vi "nanocal -- nuclear schottky fit V7.vi"() -> ()   [LabVIEW 2021] (continued)
0.000047379208   ,  \"τC\" -> 0.003106112976   ,  \"κ0\" -> 0.000000012600   ,  \"mm1\" -> 0.000044370583   ,  \"mm2\" -> 0.017847763479   ,  \"mm3\" -> 0.023626714407   ,  \"T\" -> 1.900000000000   ,  \"B\" -> 6.000000000000   ,  \"θ\" -> 0.000000000000   ,  \"Reoff\" -> -371428.571428571827   ,  \"Imoff\" -> 0.000000000000   ,  \"στ1\" -> 0.007486573720   ,  \"στS\" -> 0.000328189496   ,  \"στN\" -> 0.000005492338    |>   , \n\"IDS0454_220529_RAW_cal__sam_\" ->   <|    \"ζ\" -> 0.000000000000   ,  \"τ1\" -> 0.000000000000   ,  \"τS\" -> 0.000000000000   ,  \"τN\" -> 0.000000000000   ,  \"τC\" -> 0.000000000000   ,  \"κ0\" -> 0.000000000000   ,  \"mm1\" -> 0.000000000000   ,  \"mm2\" -> 0.000000000000   ,  \"mm3\" -> 0.000000000000   ,  \"T\" -> 1.900000000000   ,  \"B\" -> 6.000000000000   ,  \"θ\" -> 0.000000000000   ,  \"Reoff\" -> 0.000000000000   ,  \"Imoff\" -> 0.000000000000   ,  \"στ1\" -> 0.000000000000   ,  \"στS\" -> 0.000000000000   ,  \"στN\" -> 0.000000000000    |>   , \n\"IDS0455_220529_RAW_cal__ref_\" ->   <|    \"ζ\" -> 0.017684542475   ,  \"τ1\" -> 0.025415252258   ,  \"τS\" -> 0.009236528363   ,  \"τN\" -> 0.000017905293   ,  \"τC\" -> 0.002401600721   ,  \"κ0\" -> 0.000000022300   ,  \"mm1\" -> 0.000033334613   ,  \"mm2\" -> 0.011752475280   ,  \"mm3\" -> 0.025449137167   ,  \"T\" -> 3.100000000000   ,  \"B\" -> 6.000000000000   ,  \"θ\" -> 0.000000000000   ,  \"Reoff\" -> -224489.795918366871   ,  \"Imoff\" -> 0.000000000000   ,  \"στ1\" -> 0.002319336344   ,  \"στS\" -> 0.000088789026   ,  \"στN\" -> 0.000000711840    |>   , \n\"IDS0455_220529_RAW_cal__sam_\" ->   <|    \"ζ\" -> 0.000000000000   ,  \"τ1\" -> 0.000000000000   ,  \"τS\" -> 0.000000000000   ,  \"τN\" -> 0.000000000000   ,  \"τC\" -> 0.000000000000   ,  \"κ0\" -> 0.000000000000   ,  \"mm1\" -> 0.000000000000   ,  \"mm2\" -> 0.000000000000   ,  \"mm3\" -> 0.000000000000   ,  \"T\" -> 3.100000000000   ,  \"B\" -> 6.000000000000   ,  \"θ\" -> 0.000000000000   ,  \"Reoff\" -> 0.000000000000   ,  \"Imoff\" -> 0.000000000000   ,  \"στ1\" -> 0.000000000000   ,  \"στS\" -> 0.000000000000   ,  \"στN\" -> 0.000000000000    |>   , \n\"IDS0456_220529_RAW_cal__ref_\" ->   <|    \"ζ\" -> 0.018735255997   ,  \"τ1\" -> 0.025807065758   ,  \"τS\" -> 0.005944253757   ,  \"τN\" -> 0.000004775198   ,  \"τC\" -> 0.001961268842   ,  \"κ0\" -> 0.000000054800   ,  \"mm1\" -> 0.000027338307   ,  \"mm2\" -> 0.007987373292   ,  \"mm3\" -> 0.025814108537   ,  \"T\" -> 5.700000000000   ,  \"B\" -> 6.000000000000   ,  \"θ\" -> 0.000000000000   ,  \"Reoff\" -> -77551.020408162847   ,  \"Imoff\" -> 0.000000000000   ,  \"στ1\" -> 0.003676288803   ,  \"στS\" -> 0.001284267534   ,  \"στN\" -> 0.000002465031    |>   , \n\"IDS0456_220529_RAW_cal__sam_\" ->   <|    \"ζ\" -> 0.000000000000   ,  \"τ1\" -> 0.000000000000   ,  \"τS\" -> 0.000000000000   ,  \"τN\" -> 0.000000000000   ,  \"τC\" -> 0.000000000000   ,  \"κ0\" -> 0.000000000000   ,  \"mm1\" -> 0.000000000000   ,  \"mm2\" -> 0.000000000000   ,  \"mm3\" -> 0.000000000000   ,  \"T\" -> 5.700000000000   ,  \"B\" -> 6.000000000000   ,  \"θ\" -> 0.000000000000   ,  \"Reoff\" -> 0.000000000000   ,  \"Imoff\" -> 0.000000000000   ,  \"στ1\" -> 0.000000000000   ,  \"στS\" -> 0.000000000000   ,  \"στN\" -> 0.000000000000    |>   , \n\"IDS0458_220529_RAW_cal__ref_\" ->   <|    \"ζ\" -> 0.271949590763   ,  \"τ1\" -> 0.082491161116   ,  \"τS\" -> 0.016634017124   ,  \"τN\" -> 0.004711774467   ,  \"τC\" -> 0.000759404494   ,  \"κ0\" -> 0.000000000880   ,  \"mm1\" -> 0.000157873787   ,  \"mm2\" -> 0.019859290085   ,  \"mm3\" -> 0.090384172617   ,  \"T\" -> 0.200000000000   ,  \"B\" -> 4.000000000000   ,  \"θ\" -> 0.000000000000   ,  \"Reoff\" -> -53755102.040816329400   ,  \"Imoff\" -> 0.000000000000   ,  \"στ1\" -> 0.009172162575   ,  \"στS\" -> 0.000087849728   ,  \"στN\" -> 0.000215184537    |>   , \n\"IDS0458_220529_RAW_cal__sam_\" ->   <|    \"ζ\" -> 0.000000000000   ,  \"τ1\" -> 0.000000000000   ,  \"τS\" -> 0.000000000000   ,  \"τN\" -> 0.000000000000   ,  \"τC\" -> 0.000000000000   ,  \"κ0\" -> 0.000000000000   ,  \"mm1\" -> 0.000000000000   ,  \"mm2\" -> 0.000000000000   ,  \"mm3\" -> 0.000000000000   ,  \"T\" -> 0.200000000000   ,  \"B\" -> 4.000000000000   ,  \"θ\" -> 0.000000000000   ,  \"Reoff\" -> 0.000000000000   ,  \"Imoff\" -> 0.000000000000   ,  \"στ1\" -> 0.000000000000   ,  \"στS\" -> 0.000000000000   ,  \"στN\" -> 0.000000000000    |>   , \n\"IDS0459_220529_RAW_cal__ref_\" ->   <|    \"ζ\" -> 0.169028221284   ,  \"τ1\" -> 0.092219125546   ,  \"τS\" -> 0.014617231308   ,  \"τN\" -> 0.003004665048   ,  \"τC\" -> 0.000894699791   ,  \"κ0\" -> 0.000000001215   ,  \"mm1\" -> 0.000123777676   ,  \"mm2\" -> 0.017061745572   ,  \"mm3\" -> 0.096528796242   ,  \"T\" -> 0.250000000000   ,  \"B\" -> 4.000000000000   ,  \"θ\" -> 0.000000000000   ,  \"Reoff\" -> -23428571.428571432800   ,  \"Imoff\" -> 0.000000000000   ,  \"στ1\" -> 0.009019898069   ,  \"στS\" -> 0.000072357815   ,  \"στN\" -> 0.000072194130    |>   , \n\"IDS0459_220529_RAW_cal__sam_\" ->   <|    \"ζ\" -> 0.000000000000   ,  \"τ1\" -> 0.000000000000   ,  \"τS\" -> 0.000000000000   ,  \"τN\" -> 0.000000000000   ,  \"τC\" -> 0.000000000000   ,  \"κ0\" -> 0.000000000000   ,  \"mm1\" -> 0.000000000000   ,  \"mm2\" -> 0.000000000000   ,  \"mm3\" -> 0.000000000000   ,  \"T\" -> 0.250000000000   ,  \"B\" -> 4.000000000000   ,  \"θ\" -> 0.000000000000   ,  \"Reoff\" -> 0.000000000000   ,  \"Imoff\" -> 0.000000000000   ,  \"στ1\" -> 0.000000000000   ,  \"στS\" -> 0.000000000000   ,  \"στN\" -> 0.000000000000    |>   , \n\"IDS0460_220529_RAW_cal__ref_\" ->   <|    \"ζ\" -> 0.121095025204   ,  \"τ1\" -> 0.101406294737   ,  \"τS\" -> 0.013797908139   ,  \"τN\" -> 0.002167085296   ,  \"τC\" -> 0.000940421698   ,  \"κ0\" -> 0.000000001550   ,  \"mm1\" -> 0.000096322687   ,  \"mm2\" -> 0.015862507367   ,  \"mm3\" -> 0.104286161098   ,  \"T\" -> 0.300000000000   ,  \"B\" -> 4.000000000000   ,  \"θ\" -> 0.000000000000   ,  \"Reoff\" -> -14857142.857142865700   ,  \"Imoff\" -> 0.000000000000   ,  \"στ1\" -> 0.003344660593   ,  \"στS\" -> 0.000083531617   ,  \"στN\" -> 0.000031930335    |>   , \n\"IDS0460_220529_RAW_cal__sam_\" ->   <|    \"ζ\" -> 0.000000000000   ,  \"τ1\" -> 0.000000000000   ,  \"τS\" -> 0.000000000000   ,  \"τN\" -> 0.000000000000   ,  \"τC\" -> 0.000000000000   ,  \"κ0\" -> 0.000000000000   ,  \"mm1\" -> 0.000000000000   ,  \"mm2\" -> 0.000000000000   ,  \"mm3\" -> 0.000000000000   ,  \"T\" -> 0.300000000000   ,  \"B\" -> 4.000000000000   ,  \"θ\" -> 0.000000000000   ,  \"Reoff\" -> 0.000000000000   ,  \"Imoff\" -> 0.000000000000   ,  \"στ1\" -> 0.000000000000   ,  \"στS\" -> 0.000000000000   ,  \"στN\" -> 0.000000000000    |>   , \n\"IDS0461_220529_RAW_cal__ref_\" ->   <|    \"ζ\" -> 0.088720032208   ,  \"τ1\" -> 0.108699367297   ,  \"τS\" -> 0.013278602208   ,  \"τN\" -> 0.001545664659   ,  \"τC\" -> 0.001067836739   ,  \"κ0\" -> 0.000000001950   ,  \"mm1\" -> 0.000081459775   ,  \"mm2\" -> 0.015170211659   ,  \"mm3\" -> 0.110655008903   ,  \"T\" -> 0.360000000000   ,  \"B\" -> 4.000000000000   ,  \"θ\" -> 0.000000000000   ,  \"Reoff\" -> -9714285.714285701520   ,  \"Imoff\" -> 0.000000000000   ,  \"στ1\" -> 0.011282789082   ,  \"στS\" -> 0.000097113540   ,  \"στN\" -> 0.000042096921    |>   , \n\"IDS0461_220529_RAW_cal__sam_\" ->   <|    \"ζ\" -> 0.000000000000   ,  \"τ1\" -> 0.000000000000   ,  \"τS\" -> 0.000000000000   ,  \"τN\" -> 0.000000000000   ,  \"τC\" -> 0.000000000000   ,  \"κ0\" -> 0.000000000000   ,  \"mm1\" -> 0.000000000000   ,  \"mm2\" -> 0.000000000000   ,  \"mm3\" -> 0.000000000000   ,  \"T\" -> 0.360000000000   ,  \"B\" -> 4.000000000000   ,  \"θ\" -> 0.000000000000   ,  \"Reoff\" -> 0.000000000000   ,  \"Imoff\" -> 0.000000000000   ,  \"στ1\" -> 0.000000000000   ,  \"στS\" -> 0.000000000000   ,  \"στN\" -> 0.000000000000    |>   , \n\"IDS0462_220530_RAW_cal__ref_\" ->   <|    \"ζ\" -> 0.343667501463   ,  \"τ1\" -> 0.112483041616   ,  \"τS\" -> 0.019628128809   ,  \"τN\" -> 0.010154591080   ,  \"τC\" -> 0.000829297605   ,  \"κ0\" -> 0.000000000715   ,  \"mm1\" -> 0.000207215692   ,  \"mm2\" -> 0.023410434838   ,  \"mm3\" -> 0.129712761510   ,  \"T\" -> 0.170000000000   ,  \"B\" -> 4.000000000000   ,  \"θ\" -> 0.000000000000   ,  \"Reoff\" -> -62857142.857142865700   ,  \"Imoff\" -> 0.000000000000   ,  \"στ1\" -> 0.089687632936   ,  \"στS\" -> 0.000139405002   ,  \"στN\" -> 0.005363489281    |>   , \n\"IDS0462_220530_RAW_cal__sam_\" ->   <|    \"ζ\" -> 0.000000000000   ,  \"τ1\" -> 0.000000000000   ,  \"τS\" -> 0.000000000000   ,  \"τN\" -> 0.000000000000   ,  \"τC\" -> 0.000000000000   ,  \"κ0\" -> 0.000000000000   ,  \"mm1\" -> 0.000000000000   ,  \"mm2\" -> 0.000000000000   ,  \"mm3\" -> 0.000000000000   ,  \"T\" -> 0.170000000000   ,  \"B\" -> 4.000000000000   ,  \"θ\" -> 0.000000000000   ,  \"Reoff\" -> 0.000000000000   ,  \"Imoff\" -> 0.000000000000   ,  \"στ1\" -> 0.000000000000   ,  \"στS\" -> 0.000000000000   ,  \"στN\" -> 0.000000000000    |>   , \n\"IDS0463_220530_RAW_cal__ref_\" ->   <|    \"ζ\" -> 0.430227807451   ,  \"τ1\" -> 0.103641258629   ,  \"τS\" -> 0.021841444015   ,  \"τN\" -> 0.013133276363   ,  \"τC\" -> 0.000817797243   ,  \"κ0\" -> 0.000000000620   ,  \"mm1\" -> 0.000241540150   ,  \"mm2\" -> 0.025640890482   ,  \"mm3\" -> 0.128598442882   ,  \"T\" -> 0.150000000000   ,  \"B\" -> 4.000000000000   ,  \"θ\" -> 0.000000000000   ,  \"Reoff\" -> -76204081.632653057600   ,  \"Imoff\" -> 0.000000000000   ,  \"στ1\" -> 0.056966109308   ,  \"στS\" -> 0.000433843322   ,  \"στN\" -> 0.005482906809    |>   , \n\"IDS0463_220530_RAW_cal__sam_\" ->   <|    \"ζ\" -> 0.000000000000   ,  \"τ1\" -> 0.000000000000   ,  \"τS\" -> 0.000000000000   ,  \"τN\" -> 0.000000000000   ,  \"τC\" -> 0.000000000000   ,  \"κ0\" -> 0.000000000000   ,  \"mm1\" -> 0.000000000000   ,  \"mm2\" -> 0.000000000000   ,  \"mm3\" -> 0.000000000000   ,  \"T\" -> 0.150000000000   ,  \"B\" -> 4.000000000000   ,  \"θ\" -> 0.000000000000   ,  \"Reoff\" -> 0.000000000000   ,  \"Imoff\" -> 0.000000000000   ,  \"στ1\" -> 0.000000000000   ,  \"στS\" -> 0.000000000000   ,  \"στN\" -> 0.000000000000    |>   , \n\"IDS0464_220530_RAW_cal__ref_\" ->   <|    \"ζ\" -> 0.675671528717   ,  \"τ1\" -> 0.134361338288   ,  \"τS\" -> 0.029407446025   ,  \"τN\" -> 0.029781674231   ,  \"τC\" -> 0.000802871531   ,  \"κ0\" -> 0.000000000450   ,  \"mm1\" -> 0.000320592060   ,  \"mm2\" -> 0.033310531198   ,  \"mm3\" -> 0.200714610183   ,  \"T\" -> 0.120000000000   ,  \"B\" -> 4.000000000000   ,  \"θ\" -> 0.000000000000   ,  \"Reoff\" -> -173428571.428571433000   ,  \"Imoff\" -> 0.000000000000   ,  \"στ1\" -> 0.117118369535   ,  \"στS\" -> 0.002310482505   ,  \"στN\" -> 0.019921704088    |>   , \n\"IDS0464_220530_RAW_cal__sam_\" ->   <|    \"ζ\" -> 0.000000000000   ,  \"τ1\" -> 0.000000000000   ,  \"τS\" -> 0.000000000000   ,  \"τN\" -> 0.000000000000   ,  \"τC\" -> 0.000000000000   ,  \"κ0\" -> 0.000000000000   ,  \"mm1\" -> 0.000000000000   ,  \"mm2\" -> 0.000000000000   ,  \"mm3\" -> 0.000000000000   ,  \"T\" -> 0.120000000000   ,  \"B\" -> 4.000000000000   ,  \"θ\" -> 0.000000000000   ,  \"Reoff\" -> 0.000000000000   ,  \"Imoff\" -> 0.000000000000   ,  \"στ1\" -> 0.000000000000   ,  \"στS\" -> 0.000000000000   ,  \"στN\" -> 0.000000000000    |>   , \n\"IDS0465_220530_RAW_cal__ref_\" ->   <|    \"ζ\" -> 0.065985765394   ,  \"τ1\" -> 0.113805435970   ,  \"τS\" -> 0.013450011184   ,  \"τN\" -> 0.001342731867   ,  \"τC\" -> 0.001243319385   ,  \"κ0\" -> 0.000000002410   ,  \"mm1\" -> 0.000071145975   ,  \"mm2\" -> 0.015287668803   ,  \"mm3\" -> 0.115458794101   ,  \"T\" -> 0.430000000000   ,  \"B\" -> 4.000000000000   ,  \"θ\" -> 0.000000000000   ,  \"Reoff\" -> -5918367.346938773990   ,  \"Imoff\" -> 0.000000000000   ,  \"στ1\" -> 0.012030942275   ,  \"στS\" -> 0.000092415308   ,  \"στN\" -> 0.000055296571    |>   , \n\"IDS0465_220530_RAW_cal__sam_\" ->   <|    \"ζ\" -> 0.000000000000   ,  \"τ1\" -> 0.000000000000   ,  \"τS\" -> 0.000000000000   ,  \"τN\" -> 0.000000000000   ,  \"τC\" -> 0.000000000000   ,  \"κ0\" -> 0.000000000000   ,  \"mm1\" -> 0.000000000000   ,  \"mm2\" -> 0.000000000000   ,  \"mm3\" -> 0.000000000000   ,  \"T\" -> 0.430000000000   ,  \"B\" -> 4.000000000000   ,  \"θ\" -> 0.000000000000   ,  \"Reoff\" -> 0.000000000000   ,  \"Imoff\" -> 0.000000000000   ,  \"στ1\" -> 0.000000000000   ,  \"στS\" -> 0.000000000000   ,  \"στN\" -> 0.000000000000    |>   , \n\"IDS0466_220530_RAW_cal__ref_\" ->   <|    \"ζ\" -> 0.050274873948   ,  \"τ1\" -> 0.117572813394   ,  \"τS\" -> 0.013965174353   ,  \"τN\" -> 0.000622498353   ,  \"τC\" -> 0.001752185729   ,  \"κ0\" -> 0.000000003045   ,  \"mm1\" -> 0.000075268427   ,  \"mm2\" -> 0.016239468880   ,  \"mm3\" -> 0.118331327928   ,  \"T\" -> 0.530000000000   ,  \"B\" -> 4.000000000000   ,  \"θ\" -> 0.000000000000   ,  \"Reoff\" -> -3204081.632653061300   ,  \"Imoff\" -> 0.000000000000   ,  \"στ1\" -> 0.009611649331   ,  \"στS\" -> 0.000172547734   ,  \"στN\" -> 0.000019241473    |>   , \n\"IDS0466_220530_RAW_cal__sam_\" ->   <|    \"ζ\" -> 0.000000000000   ,  \"τ1\" -> 0.000000000000   ,  \"τS\" -> 0.000000000000   ,  \"τN\" -> 0.000000000000   ,  \"τC\" -> 0.000000000000   ,  \"κ0\" -> 0.000000000000   ,  \"mm1\" -> 0.000000000000   ,  \"mm2\" -> 0.000000000000   ,  \"mm3\" -> 0.000000000000   ,  \"T\" -> 0.530000000000   ,  \"B\" -> 4.000000000000   ,  \"θ\" -> 0.000000000000   ,  \"Reoff\" -> 0.000000000000   ,  \"Imoff\" -> 0.000000000000   ,  \"στ1\" -> 0.000000000000   ,  \"στS\" -> 0.000000000000   ,  \"στN\" -> 0.000000000000    |>   , \n\"IDS0467_220530_RAW_cal__ref_\" ->   <|    \"ζ\" -> 0.041054990767   ,  \"τ1\" -> 0.119173098156   ,  \"τS\" -> 0.015405145420   ,  \"τN\" -> 0.000278319894   ,  \"τC\" -> 0.001789500233   ,  \"κ0\" -> 0.000000003708   ,  \"mm1\" -> 0.000063714353   ,  \"mm2\" -> 0.017712825393   ,  \"mm3\" -> 0.119513408481   ,  \"T\" -> 0.620000000000   ,  \"B\" -> 4.000000000000   ,  \"θ\" -> 0.000000000000   ,  \"Reoff\" -> -2755102.040816326160   ,  \"Imoff\" -> 0.000000000000   ,  \"στ1\" -> 0.018149556060   ,  \"στS\" -> 0.000211563346   ,  \"στN\" -> 0.000013374065    |>   , \n\"IDS0467_220530_RAW_cal__sam_\" ->   <|    \"ζ\" -> 0.000000000000   ,  \"τ1\" -> 0.000000000000   ,  \"τS\" -> 0.000000000000   ,  \"τN\" -> 0.000000000000   ,  \"τC\" -> 0.000000000000   ,  \"κ0\" -> 0.000000000000   ,  \"mm1\" -> 0.000000000000   ,  \"mm2\" -> 0.000000000000   ,  \"mm3\" -> 0.000000000000   ,  \"T\" -> 0.620000000000   ,  \"B\" -> 4.000000000000   ,  \"θ\" -> 0.000000000000   ,  \"Reoff\" -> 0.000000000000   ,  \"Imoff\" -> 0.000000000000   ,  \"στ1\" -> 0.000000000000   ,  \"στS\" -> 0.000000000000   ,  \"στN\" -> 0.000000000000    |>   , \n\"IDS0468_220530_RAW_cal__ref_\" ->   <|    \"ζ\" -> 0.028502781656   ,  \"τ1\" -> 0.123145264277   ,  \"τS\" -> 0.019280232525   ,  \"τN\" -> 0.000154237911   ,  \"τC\" -> 0.002123664207   ,  \"κ0\" -> 0.000000005085   ,  \"mm1\" -> 0.000053289074   ,  \"mm2\" -> 0.021865908006   ,  \"mm3\" -> 0.123338138308   ,  \"T\" -> 0.820000000000   ,  \"B\" -> 4.000000000000   ,  \"θ\" -> 0.000000000000   ,  \"Reoff\" -> -1265306.122448980810   ,  \"Imoff\" -> 0.000000000000   ,  \"στ1\" -> 0.018340702428   ,  \"στS\" -> 0.000185539060   ,  \"στN\" -> 0.000003670517    |>   , \n\"IDS0468_220530_RAW_cal__sam_\" ->   <|    \"ζ\" -> 0.000000000000   ,  \"τ1\" -> 0.000000000000   ,  \"τS\" -> 0.000000000000   ,  \"τN\" -> 0.000000000000   ,  \"τC\" -> 0.000000000000   ,  \"κ0\" -> 0.000000000000   ,  \"mm1\" -> 0.000000000000   ,  \"mm2\" -> 0.000000000000   ,  \"mm3\" -> 0.000000000000   ,  \"T\" -> 0.820000000000   ,  \"B\" -> 4.000000000000   ,  \"θ\" -> 0.000000000000   ,  \"Reoff\" -> 0.000000000000   ,  \"Imoff\" -> 0.000000000000   ,  \"στ1\" -> 0.000000000000   ,  \"στS\" -> 0.000000000000   ,  \"στN\" -> 0.000000000000    |>   , \n\"IDS0469_220530_RAW_cal__ref_\" ->   <|    \"ζ\" -> 0.021661724597   ,  \"τ1\" -> 0.135376034198   ,  \"τS\" -> 0.027370656195   ,  \"τN\" -> 0.000065416524   ,  \"τC\" -> 0.002262892828   ,  \"κ0\" -> 0.000000007163   ,  \"mm1\" -> 0.000044452306   ,  \"mm2\" -> 0.030162834530   ,  \"mm3\" -> 0.135462025560   ,  \"T\" -> 1.120000000000   ,  \"B\" -> 4.000000000000   ,  \"θ\" -> 0.000000000000   ,  \"Reoff\" -> -775510.204081632196   ,  \"Imoff\" -> 0.000000000000   ,  \"στ1\" -> 0.011862460543   ,  \"στS\" -> 0.000298822899   ,  \"στN\" -> 0.000002245413    |>   , \n\"IDS0469_220530_RAW_cal__sam_\" ->   <|    \"ζ\" -> 0.000000000000   ,  \"τ1\" -> 0.000000000000   ,  \"τS\" -> 0.000000000000   ,  \"τN\" -> 0.000000000000   ,  \"τC\" -> 0.000000000000   ,  \"κ0\" -> 0.000000000000   ,  \"mm1\" -> 0.000000000000   ,  \"mm2\" -> 0.000000000000   ,  \"mm3\" -> 0.000000000000   ,  \"T\" -> 1.120000000000   ,  \"B\" -> 4.000000000000   ,  \"θ\" -> 0.000000000000   ,  \"Reoff\" -> 0.000000000000   ,  \"Imoff\" -> 0.000000000000   ,  \"στ1\" -> 0.000000000000   ,  \"στS\" -> 0.000000000000   ,  \"στN\" -> 0.000000000000    |>   , \n\"IDS0470_220530_RAW_cal__ref_\" ->   <|    \"ζ\" -> 0.015441202200   ,  \"τ1\" -> 0.041977704334   ,  \"τS\" -> 0.036507196019   ,  \"τN\" -> 0.000016236903   ,  \"τC\" -> 0.002199544538   ,  \"κ0\" -> 0.000000012895   ,  \"mm1\" -> 0.000031599194   ,  \"mm2\" -> 0.039021251943   ,  \"mm3\" -> 0.042211796370   ,  \"T\" -> 1.900000000000   ,  \"B\" -> 4.000000000000   ,  \"θ\" -> 0.000000000000   ,  \"Reoff\" -> -265306.122448978945   ,  \"Imoff\" -> 0.000000000000   ,  \"στ1\" -> 0.036878491395   ,  \"στS\" -> 0.000608860312   ,  \"στN\" -> 0.000004645190    |>   , \n\"IDS0470_220530_RAW_cal__sam_\" ->   <|    \"ζ\" -> 0.000000000000   ,  \"τ1\" -> 0.000000000000   ,  \"τS\" -> 0.000000000000   ,  \"τN\" -> 0.000000000000   ,  \"τC\" -> 0.000000000000   ,  \"κ0\" -> 0.000000000000   ,  \"mm1\" -> 0.000000000000   ,  \"mm2\" -> 0.000000000000   ,  \"mm3\" -> 0.000000000000   ,  \"T\" -> 1.900000000000   ,  \"B\" -> 4.000000000000   ,  \"θ\" -> 0.000000000000   ,  \"Reoff\" -> 0.000000000000   ,  \"Imoff\" -> 0.000000000000   ,  \"στ1\" -> 0.000000000000   ,  \"στS\" -> 0.000000000000   ,  \"στN\" -> 0.000000000000    |>   , \n\"IDS0471_220530_RAW_cal__ref_\" ->   <|    \"ζ\" -> 0.014899977348   ,  \"τ1\" -> 0.039852327400   ,  \"τS\" -> 0.012042479771   ,  \"τN\" -> 0.000007668254   ,  \"τC\" -> 0.002248141599   ,  \"κ0\" -> 0.000000015723   ,  \"mm1\" -> 0.000027931492   ,  \"mm2\" -> 0.014437702970   ,  \"mm3\" -> 0.039864529495   ,  \"T\" -> 2.300000000000   ,  \"B\" -> 4.000000000000   ,  \"θ\" -> 0.000000000000   ,  \"Reoff\" -> -183673.469387754798   ,  \"Imoff\" -> 0.000000000000   ,  \"στ1\" -> 0.000774965788   ,  \"στS\" -> 0.000109876194   ,  \"στN\" -> 0.000000141932    |>   , \n\"IDS0471_220530_RAW_cal__sam_\" ->   <|    \"ζ\" -> 0.000000000000   ,  \"τ1\" -> 0.000000000000   ,  \"τS\" -> 0.000000000000   ,  \"τN\" -> 0.000000000000   ,  \"τC\" -> 0.000000000000   ,  \"κ0\" -> 0.000000000000   ,  \"mm1\" -> 0.000000000000   ,  \"mm2\" -> 0.000000000000   ,  \"mm3\" -> 0.000000000000   ,  \"T\" -> 2.300000000000   ,  \"B\" -> 4.000000000000   ,  \"θ\" -> 0.000000000000   ,  \"Reoff\" -> 0.000000000000   ,  \"Imoff\" -> 0.000000000000   ,  \"στ1\" -> 0.000000000000   ,  \"στS\" -> 0.000000000000   ,  \"στN\" -> 0.000000000000    |>   , \n\"IDS0472_220530_RAW_cal__ref_\" ->   <|    \"ζ\" -> 0.016604913016   ,  \"τ1\" -> 0.039295846672   ,  \"τS\" -> 0.009676137271   ,  \"τN\" -> 0.000004030512   ,  \"τC\" -> 0.002212920920   ,  \"κ0\" -> 0.000000022506   ,  \"mm1\" -> 0.000029579758   ,  \"mm2\" -> 0.012018345525   ,  \"mm3\" -> 0.039301748436   ,  \"T\" -> 3.070000000000   ,  \"B\" -> 4.000000000000   ,  \"θ\" -> 0.000000000000   ,  \"Reoff\" -> -183673.469387754798   ,  \"Imoff\" -> 0.000000000000   ,  \"στ1\" -> 0.024245559529   ,  \"στS\" -> 0.008314224018   ,  \"στN\" -> 0.000009266489    |>   , \n\"IDS0472_220530_RAW_cal__sam_\" ->   <|    \"ζ\" -> 0.000000000000   ,  \"τ1\" -> 0.000000000000   ,  \"τS\" -> 0.000000000000   ,  \"τN\" -> 0.000000000000   ,  \"τC\" -> 0.000000000000   ,  \"κ0\" -> 0.000000000000   ,  \"mm1\" -> 0.000000000000   ,  \"mm2\" -> 0.000000000000   ,  \"mm3\" -> 0.000000000000   ,  \"T\" -> 3.070000000000   ,  \"B\" -> 4.000000000000   ,  \"θ\" -> 0.000000000000   ,  \"Reoff\" -> 0.000000000000   ,  \"Imoff\" -> 0.000000000000   ,  \"στ1\" -> 0.000000000000   ,  \"στS\" -> 0.000000000000   ,  \"στN\" -> 0.000000000000    |>   , \n\"IDS0473_220531_RAW_cal__ref_\" ->   <|    \"ζ\" -> 0.018700689738   ,  \"τ1\" -> 0.039247142341   ,  \"τS\" -> 0.006094502124   ,  \"τN\" -> 0.000001379348   ,  \"τC\" -> 0.001765569741   ,  \"κ0\" -> 0.000000055137   ,  \"mm1\" -> 0.000025315301   ,  \"mm2\" -> 0.007948371438   ,  \"mm3\" -> 0.039248904003   ,  \"T\" -> 5.700000000000   ,  \"B\" -> 4.000000000000   ,  \"θ\" -> 0.000000000000   ,  \"Reoff\" -> -102040.816326530650   ,  \"Imoff\" -> 0.000000000000   ,  \"στ1\" -> 0.006123782667   ,  \"στS\" -> 0.001309533453   ,  \"στN\" -> 0.000000787923    |>   , \n\"IDS0473_220531_RAW_cal__sam_\" ->   <|    \"ζ\" -> 0.000000000000   ,  \"τ1\" -> 0.000000000000   ,  \"τS\" -> 0.000000000000   ,  \"τN\" -> 0.000000000000   ,  \"τC\" -> 0.000000000000   ,  \"κ0\" -> 0.000000000000   ,  \"mm1\" -> 0.000000000000   ,  \"mm2\" -> 0.000000000000   ,  \"mm3\" -> 0.000000000000   ,  \"T\" -> 5.700000000000   ,  \"B\" -> 4.000000000000   ,  \"θ\" -> 0.000000000000   ,  \"Reoff\" -> 0.000000000000   ,  \"Imoff\" -> 0.000000000000   ,  \"στ1\" -> 0.000000000000   ,  \"στS\" -> 0.000000000000   ,  \"στN\" -> 0.000000000000    |>   , \n\"IDS0477_220601_RAW_cal__ref_\" ->   <|    \"ζ\" -> 0.239805642697   ,  \"τ1\" -> 0.033790664831   ,  \"τS\" -> 0.059024379220   ,  \"τN\" -> 0.060427064379   ,  \"τC\" -> 0.000896937980   ,  \"κ0\" -> 0.000000000920   ,  \"mm1\" -> 0.000171776345   ,  \"mm2\" -> 0.014890032084   ,  \"mm3\" -> 0.167722368184   ,  \"T\" -> 0.200000000000   ,  \"B\" -> 10.000000000000   ,  \"θ\" -> 45.000000000000   ,  \"Reoff\" -> -36122448.979591839000   ,  \"Imoff\" -> 0.000000000000   ,  \"στ1\" -> 0.011907202865   ,  \"στS\" -> 0.006392080806   ,  \"στN\" -> 0.010956766376    |>   , \n\"IDS0477_220601_RAW_cal__sam_\" ->   <|    \"ζ\" -> 0.000000000000   ,  \"τ1\" -> 0.000000000000   ,  \"τS\" -> 0.000000000000   ,  \"τN\" -> 0.000000000000   ,  \"τC\" -> 0.000000000000   ,  \"κ0\" -> 0.000000000000   ,  \"mm1\" -> 0.000000000000   ,  \"mm2\" -> 0.000000000000   ,  \"mm3\" -> 0.000000000000   ,  \"T\" -> 0.200000000000   ,  \"B\" -> 10.000000000000   ,  \"θ\" -> 45.000000000000   ,  \"Reoff\" -> 0.000000000000   ,  \"Imoff\" -> 0.000000000000   ,  \"στ1\" -> 0.000000000000   ,  \"στS\" -> 0.000000000000   ,  \"στN\" -> 0.000000000000    |>   , \n\"IDS0478_220601_RAW_cal__ref_\" ->   <|    \"ζ\" -> 0.152803180528   ,  \"τ1\" -> 0.028187868792   ,  \"τS\" -> 0.047098340694   ,  \"τN\" -> 0.025207837056   ,  \"τC\" -> 0.000982024605   ,  \"κ0\" -> 0.000000001260   ,  \"mm1\" -> 0.000128146365   ,  \"mm2\" -> 0.016152622122   ,  \"mm3\" -> 0.096243916593   ,  \"T\" -> 0.250000000000   ,  \"B\" -> 10.000000000000   ,  \"θ\" -> 45.000000000000   ,  \"Reoff\" -> -18163265.306122452000   ,  \"Imoff\" -> 0.000000000000   ,  \"στ1\" -> 0.005041045857   ,  \"στS\" -> 0.001567344139   ,  \"στN\" -> 0.002277988599    |>   , \n\"IDS0478_220601_RAW_cal__sam_\" ->   <|    \"ζ\" -> 0.000000000000   ,  \"τ1\" -> 0.000000000000   ,  \"τS\" -> 0.000000000000   ,  \"τN\" -> 0.000000000000   ,  \"τC\" -> 0.000000000000   ,  \"κ0\" -> 0.000000000000   ,  \"mm1\" -> 0.000000000000   ,  \"mm2\" -> 0.000000000000   ,  \"mm3\" -> 0.000000000000   ,  \"T\" -> 0.250000000000   ,  \"B\" -> 10.000000000000   ,  \"θ\" -> 45.000000000000   ,  \"Reoff\" -> 0.000000000000   ,  \"Imoff\" -> 0.000000000000   ,  \"στ1\" -> 0.000000000000   ,  \"στS\" -> 0.000000000000   ,  \"στN\" -> 0.000000000000    |>   , \n\"IDS0479_220601_RAW_cal__ref_\" ->   <|    \"ζ\" -> 0.111193066205   ,  \"τ1\" -> 0.024122553376   ,  \"τS\" -> 0.042118651402   ,  \"τN\" -> 0.013651970206   ,  \"τC\" -> 0.001072327817   ,  \"κ0\" -> 0.000000001570   ,  \"mm1\" -> 0.000105128315   ,  \"mm2\" -> 0.016280391263   ,  \"mm3\" -> 0.070781289644   ,  \"T\" -> 0.300000000000   ,  \"B\" -> 10.000000000000   ,  \"θ\" -> 45.000000000000   ,  \"Reoff\" -> -10816326.530612245200   ,  \"Imoff\" -> 0.000000000000   ,  \"στ1\" -> 0.003531051170   ,  \"στS\" -> 0.000678989919   ,  \"στN\" -> 0.000877996668    |>   , \n\"IDS0479_220601_RAW_cal__sam_\" ->   <|    \"ζ\" -> 0.000000000000   ,  \"τ1\" -> 0.000000000000   ,  \"τS\" -> 0.000000000000   ,  \"τN\" -> 0.000000000000   ,  \"τC\" -> 0.000000000000   ,  \"κ0\" -> 0.000000000000   ,  \"mm1\" -> 0.000000000000   ,  \"mm2\" -> 0.000000000000   ,  \"mm3\" -> 0.000000000000   ,  \"T\" -> 0.300000000000   ,  \"B\" -> 10.000000000000   ,  \"θ\" -> 45.000000000000   ,  \"Reoff\" -> 0.000000000000   ,  \"Imoff\" -> 0.000000000000   ,  \"στ1\" -> 0.000000000000   ,  \"στS\" -> 0.000000000000   ,  \"στN\" -> 0.000000000000    |>   , \n\"IDS0480_220601_RAW_cal__ref_\" ->   <|    \"ζ\" -> 0.079231560459   ,  \"τ1\" -> 0.017107381840   ,  \"τS\" -> 0.036891145607   ,  \"τN\" -> 0.007202328301   ,  \"τC\" -> 0.001264563258   ,  \"κ0\" -> 0.000000002000   ,  \"mm1\" -> 0.000090175019   ,  \"mm2\" -> 0.013352548983   ,  \"mm3\" -> 0.052516289748   ,  \"T\" -> 0.360000000000   ,  \"B\" -> 10.000000000000   ,  \"θ\" -> 45.000000000000   ,  \"Reoff\" -> -6326530.612244904040   ,  \"Imoff\" -> 0.000000000000   ,  \"στ1\" -> 0.001933309697   ,  \"στS\" -> 0.000284795622   ,  \"στN\" -> 0.000344056722    |>   , \n\"IDS0480_220601_RAW_cal__sam_\" ->   <|    \"ζ\" -> 0.000000000000   ,  \"τ1\" -> 0.000000000000   ,  \"τS\" -> 0.000000000000   ,  \"τN\" -> 0.000000000000   ,  \"τC\" -> 0.000000000000   ,  \"κ0\" -> 0.000000000000   ,  \"mm1\" -> 0.000000000000   ,  \"mm2\" -> 0.000000000000   ,  \"mm3\" -> 0.000000000000   ,  \"T\" -> 0.360000000000   ,  \"B\" -> 10.000000000000   ,  \"θ\" -> 45.000000000000   ,  \"Reoff\" -> 0.000000000000   ,  \"Imoff\" -> 0.000000000000   ,  \"στ1\" -> 0.000000000000   ,  \"στS\" -> 0.000000000000   ,  \"στN\" -> 0.000000000000    |>   , \n\"IDS0481_220601_RAW_cal__ref_\" ->   <|    \"ζ\" -> 0.059346185114   ,  \"τ1\" -> 0.015969775027   ,  \"τS\" -> 0.034144098652   ,  \"τN\" -> 0.004294468384   ,  \"τC\" -> 0.001604549811   ,  \"κ0\" -> 0.000000002410   ,  \"mm1\" -> 0.000086265768   ,  \"mm2\" -> 0.013446939913   ,  \"mm3\" -> 0.044760868507   ,  \"T\" -> 0.420000000000   ,  \"B\" -> 10.000000000000   ,  \"θ\" -> 45.000000000000   ,  \"Reoff\" -> -3061224.489795923230   ,  \"Imoff\" -> 0.000000000000   ,  \"στ1\" -> 0.000907344416   ,  \"στS\" -> 0.000176030005   ,  \"στN\" -> 0.000148751487    |>   , \n\"IDS0481_220601_RAW_cal__sam_\" ->   <|    \"ζ\" -> 0.000000000000   ,  \"τ1\" -> 0.000000000000   ,  \"τS\" -> 0.000000000000   ,  \"τN\" -> 0.000000000000   ,  \"τC\" -> 0.000000000000   ,  \"κ0\" -> 0.000000000000   ,  \"mm1\" -> 0.000000000000   ,  \"mm2\" -> 0.000000000000   ,  \"mm3\" -> 0.000000000000   ,  \"T\" -> 0.420000000000   ,  \"B\" -> 10.000000000000   ,  \"θ\" -> 45.000000000000   ,  \"Reoff\" -> 0.000000000000   ,  \"Imoff\" -> 0.000000000000   ,  \"στ1\" -> 0.000000000000   ,  \"στS\" -> 0.000000000000   ,  \"στN\" -> 0.000000000000    |>   , \n\"IDS0482_220601_RAW_cal__ref_\" ->   <|    \"ζ\" -> 0.043142553496   ,  \"τ1\" -> 0.014499389185   ,  \"τS\" -> 0.030371945733   ,  \"τN\" -> 0.002402650316   ,  \"τC\" -> 0.001877907190   ,  \"κ0\" -> 0.000000003100   ,  \"mm1\" -> 0.000073480289   ,  \"mm2\" -> 0.012924539137   ,  \"mm3\" -> 0.037567852762   ,  \"T\" -> 0.520000000000   ,  \"B\" -> 10.000000000000   ,  \"θ\" -> 45.000000000000   ,  \"Reoff\" -> -1836734.693877555430   ,  \"Imoff\" -> 0.000000000000   ,  \"στ1\" -> 0.000488095502   ,  \"στS\" -> 0.000097405917   ,  \"στN\" -> 0.000051506778    |>   , \n\"IDS0482_220601_RAW_cal__sam_\" ->   <|    \"ζ\" -> 0.000000000000   ,  \"τ1\" -> 0.000000000000   ,  \"τS\" -> 0.000000000000   ,  \"τN\" -> 0.000000000000   ,  \"τC\" -> 0.000000000000   ,  \"κ0\" -> 0.000000000000   ,  \"mm1\" -> 0.000000000000   ,  \"mm2\" -> 0.000000000000   ,  \"mm3\" -> 0.000000000000   ,  \"T\" -> 0.520000000000   ,  \"B\" -> 10.000000000000   ,  \"θ\" -> 45.000000000000   ,  \"Reoff\" -> 0.000000000000   ,  \"Imoff\" -> 0.000000000000   ,  \"στ1\" -> 0.000000000000   ,  \"στS\" -> 0.000000000000   ,  \"στN\" -> 0.000000000000    |>   , \n\"IDS0483_220601_RAW_cal__ref_\" ->   <|    \"ζ\" -> 0.037957534412   ,  \"τ1\" -> 0.013025982486   ,  \"τS\" -> 0.027861955043   ,  \"τN\" -> 0.001482537125   ,  \"τC\" -> 0.001562153050   ,  \"κ0\" -> 0.000000003750   ,  \"mm1\" -> 0.000054295490   ,  \"mm2\" -> 0.012021211304   ,  \"mm3\" -> 0.032970965481   ,  \"T\" -> 0.620000000000   ,  \"B\" -> 10.000000000000   ,  \"θ\" -> 45.000000000000   ,  \"Reoff\" -> -2489795.918367348610   ,  \"Imoff\" -> 0.000000000000   ,  \"στ1\" -> 0.000872811735   ,  \"στS\" -> 0.000114206450   ,  \"στN\" -> 0.000055407234    |>   , \n\"IDS0483_220601_RAW_cal__sam_\" ->   <|    \"ζ\" -> 0.000000000000   ,  \"τ1\" -> 0.000000000000   ,  \"τS\" -> 0.000000000000   ,  \"τN\" -> 0.000000000000   ,  \"τC\" -> 0.000000000000   ,  \"κ0\" -> 0.000000000000   ,  \"mm1\" -> 0.000000000000   ,  \"mm2\" -> 0.000000000000   ,  \"mm3\" -> 0.000000000000   ,  \"T\" -> 0.620000000000   ,  \"B\" -> 10.000000000000   ,  \"θ\" -> 45.000000000000   ,  \"Reoff\" -> 0.000000000000   ,  \"Imoff\" -> 0.000000000000   ,  \"στ1\" -> 0.000000000000   ,  \"στS\" -> 0.000000000000   ,  \"στN\" -> 0.000000000000    |>   , \n\"IDS0484_220601_RAW_cal__ref_\" ->   <|    \"ζ\" -> 0.026779879048   ,  \"τ1\" -> 0.012724854717   ,  \"τS\" -> 0.023406495826   ,  \"τN\" -> 0.000845574693   ,  \"τC\" -> 0.002190018434   ,  \"κ0\" -> 0.000000005114   ,  \"mm1\" -> 0.000052452848   ,  \"mm2\" -> 0.011990951083   ,  \"mm3\" -> 0.027773007254   ,  \"T\" -> 0.820000000000   ,  \"B\" -> 10.000000000000   ,  \"θ\" -> 45.000000000000   ,  \"Reoff\" -> -1020408.163265310230   ,  \"Imoff\" -> 0.000000000000   ,  \"στ1\" -> 0.000585844678   ,  \"στS\" -> 0.000123901377   ,  \"στN\" -> 0.000022627070    |>   , \n\"IDS0484_220601_RAW_cal__sam_\" ->   <|    \"ζ\" -> 0.000000000000   ,  \"τ1\" -> 0.000000000000   ,  \"τS\" -> 0.000000000000   ,  \"τN\" -> 0.000000000000   ,  \"τC\" -> 0.000000000000   ,  \"κ0\" -> 0.000000000000   ,  \"mm1\" -> 0.000000000000   ,  \"mm2\" -> 0.000000000000   ,  \"mm3\" -> 0.000000000000   ,  \"T\" -> 0.820000000000   ,  \"B\" -> 10.000000000000   ,  \"θ\" -> 45.000000000000   ,  \"Reoff\" -> 0.000000000000   ,  \"Imoff\" -> 0.000000000000   ,  \"στ1\" -> 0.000000000000   ,  \"στS\" -> 0.000000000000   ,  \"στN\" -> 0.000000000000    |>   , \n\"IDS0485_220601_RAW_cal__ref_\" ->   <|    \"ζ\" -> 0.326622885443   ,  \"τ1\" -> 0.044212332753   ,  \"τS\" -> 0.078119393187   ,  \"τN\" -> 0.109436103453   ,  \"τC\" -> 0.000856629079   ,  \"κ0\" -> 0.000000000725   ,  \"mm1\" -> 0.000209590105   ,  \"mm2\" -> 0.016643396508   ,  \"mm3\" -> 0.277031389353   ,  \"T\" -> 0.170000000000   ,  \"B\" -> 10.000000000000   ,  \"θ\" -> 45.000000000000   ,  \"Reoff\" -> -62040816.326530613000   ,  \"Imoff\" -> 0.000000000000   ,  \"στ1\" -> 0.024054965225   ,  \"στS\" -> 0.017110063636   ,  \"στN\" -> 0.032486922745    |>   , \n\"IDS0485_220601_RAW_cal__sam_\" ->   <|    \"ζ\" -> 0.000000000000   ,  \"τ1\" -> 0.000000000000   ,  \"τS\" -> 0.000000000000   ,  \"τN\" -> 0.000000000000   ,  \"τC\" -> 0.000000000000   ,  \"κ0\" -> 0.000000000000   ,  \"mm1\" -> 0.000000000000   ,  \"mm2\" -> 0.000000000000   ,  \"mm3\" -> 0.000000000000   ,  \"T\" -> 0.170000000000   ,  \"B\" -> 10.000000000000   ,  \"θ\" -> 45.000000000000   ,  \"Reoff\" -> 0.000000000000   ,  \"Imoff\" -> 0.000000000000   ,  \"στ1\" -> 0.000000000000   ,  \"στS\" -> 0.000000000000   ,  \"στN\" -> 0.000000000000    |>   , \n\"IDS0486_220602_RAW_cal__ref_\" ->   <|    \"ζ\" -> 0.647357967210   ,  \"τ1\" -> 0.057848718155   ,  \"τS\" -> 0.135216834392   ,  \"τN\" -> 0.439833290844   ,  \"τC\" -> 0.000803496040   ,  \"κ0\" -> 0.000000000457   ,  \"mm1\" -> 0.000315044381   ,  \"mm2\" -> 0.013010354662   ,  \"mm3\" -> 0.992640220504   ,  \"T\" -> 0.120000000000   ,  \"B\" -> 10.000000000000   ,  \"θ\" -> 45.000000000000   ,  \"Reoff\" -> -171836734.693877578000   ,  \"Imoff\" -> 0.000000000000   ,  \"στ1\" -> 0.042149570105   ,  \"στS\" -> 0.062954836972   ,  \"στN\" -> 0.160749966190    |>   , \n\"IDS0486_220602_RAW_cal__sam_\" ->   <|    \"ζ\" -> 0.000000000000   ,  \"τ1\" -> 0.000000000000   ,  \"τS\" -> 0.000000000000   ,  \"τN\" -> 0.000000000000   ,  \"τC\" -> 0.000000000000   ,  \"κ0\" -> 0.000000000000   ,  \"mm1\" -> 0.000000000000   ,  \"mm2\" -> 0.000000000000   ,  \"mm3\" -> 0.000000000000   ,  \"T\" -> 0.120000000000   ,  \"B\" -> 10.000000000000   ,  \"θ\" -> 45.000000000000   ,  \"Reoff\" -> 0.000000000000   ,  \"Imoff\" -> 0.000000000000   ,  \"στ1\" -> 0.000000000000   ,  \"στS\" -> 0.000000000000   ,  \"στN\" -> 0.000000000000    |>   , \n\"IDS0487_220602_RAW_cal__ref_\" ->   <|    \"ζ\" -> 0.413977366659   ,  \"τ1\" -> 0.044491025512   ,  \"τS\" -> 0.091456784931   ,  \"τN\" -> 0.162770283044   ,  \"τC\" -> 0.000783758784   ,  \"κ0\" -> 0.000000000637   ,  \"mm1\" -> 0.000228474902   ,  \"mm2\" -> 0.014828264072   ,  \"mm3\" -> 0.389689365431   ,  \"T\" -> 0.150000000000   ,  \"B\" -> 10.000000000000   ,  \"θ\" -> 45.000000000000   ,  \"Reoff\" -> -87632653.061224490400   ,  \"Imoff\" -> 0.000000000000   ,  \"στ1\" -> 0.020687994730   ,  \"στS\" -> 0.021344943576   ,  \"στN\" -> 0.040787910782    |>   , \n\"IDS0487_220602_RAW_cal__sam_\" ->   <|    \"ζ\" -> 0.000000000000   ,  \"τ1\" -> 0.000000000000   ,  \"τS\" -> 0.000000000000   ,  \"τN\" -> 0.000000000000   ,  \"τC\" -> 0.000000000000   ,  \"κ0\" -> 0.000000000000   ,  \"mm1\" -> 0.000000000000   ,  \"mm2\" -> 0.000000000000   ,  \"mm3\" -> 0.000000000000   ,  \"T\" -> 0.150000000000   ,  \"B\" -> 10.000000000000   ,  \"θ\" -> 45.000000000000   ,  \"Reoff\" -> 0.000000000000   ,  \"Imoff\" -> 0.000000000000   ,  \"στ1\" -> 0.000000000000   ,  \"στS\" -> 0.000000000000   ,  \"στN\" -> 0.000000000000    |>   , \n\"IDS0488_220602_RAW_cal__ref_\" ->   <|    \"ζ\" -> 0.022173506919   ,  \"τ1\" -> 0.011885040231   ,  \"τS\" -> 0.019213986471   ,  \"τN\" -> 0.000342476634   ,  \"τC\" -> 0.002250605678   ,  \"κ0\" -> 0.000000007250   ,  \"mm1\" -> 0.000043889604   ,  \"mm2\" -> 0.011496376729   ,  \"mm3\" -> 0.022585478052   ,  \"T\" -> 1.120000000000   ,  \"B\" -> 10.000000000000   ,  \"θ\" -> 45.000000000000   ,  \"Reoff\" -> -775510.204081632196   ,  \"Imoff\" -> 0.000000000000   ,  \"στ1\" -> 0.000592033773   ,  \"στS\" -> 0.000127596201   ,  \"στN\" -> 0.000006161863    |>   , \n\"IDS0488_220602_RAW_cal__sam_\" ->   <|    \"ζ\" -> 0.000000000000   ,  \"τ1\" -> 0.000000000000   ,  \"τS\" -> 0.000000000000   ,  \"τN\" -> 0.000000000000   ,  \"τC\" -> 0.000000000000   ,  \"κ0\" -> 0.000000000000   ,  \"mm1\" -> 0.000000000000   ,  \"mm2\" -> 0.000000000000   ,  \"mm3\" -> 0.000000000000   ,  \"T\" -> 1.120000000000   ,  \"B\" -> 10.000000000000   ,  \"θ\" -> 45.000000000000   ,  \"Reoff\" -> 0.000000000000   ,  \"Imoff\" -> 0.000000000000   ,  \"στ1\" -> 0.000000000000   ,  \"στS\" -> 0.000000000000   ,  \"στN\" -> 0.000000000000    |>   , \n\"IDS0489_220602_RAW_cal__ref_\" ->   <|    \"ζ\" -> 0.017747577510   ,  \"τ1\" -> 0.012094843134   ,  \"τS\" -> 0.012989013001   ,  \"τN\" -> 0.000085603032   ,  \"τC\" -> 0.003089605627   ,  \"κ0\" -> 0.000000012681   ,  \"mm1\" -> 0.000043787767   ,  \"mm2\" -> 0.011860461021   ,  \"mm3\" -> 0.016586858767   ,  \"T\" -> 1.900000000000   ,  \"B\" -> 10.000000000000   ,  \"θ\" -> 45.000000000000   ,  \"Reoff\" -> -285714.285714283585   ,  \"Imoff\" -> 0.000000000000   ,  \"στ1\" -> 0.000492222129   ,  \"στS\" -> 0.000068169784   ,  \"στN\" -> 0.000002379689    |>   , \n\"IDS0489_220602_RAW_cal__sam_\" ->   <|    \"ζ\" -> 0.000000000000   ,  \"τ1\" -> 0.000000000000   ,  \"τS\" -> 0.000000000000   ,  \"τN\" -> 0.000000000000   ,  \"τC\" -> 0.000000000000   ,  \"κ0\" -> 0.000000000000   ,  \"mm1\" -> 0.000000000000   ,  \"mm2\" -> 0.000000000000   ,  \"mm3\" -> 0.000000000000   ,  \"T\" -> 1.900000000000   ,  \"B\" -> 10.000000000000   ,  \"θ\" -> 45.000000000000   ,  \"Reoff\" -> 0.000000000000   ,  \"Imoff\" -> 0.000000000000   ,  \"στ1\" -> 0.000000000000   ,  \"στS\" -> 0.000000000000   ,  \"στN\" -> 0.000000000000    |>   , \n\"IDS0490_220602_RAW_cal__ref_\" ->   <|    \"ζ\" -> 0.017719366864   ,  \"τ1\" -> 0.012304843107   ,  \"τS\" -> 0.009230373075   ,  \"τN\" -> 0.000023645241   ,  \"τC\" -> 0.002722388049   ,  \"κ0\" -> 0.000000022572   ,  \"mm1\" -> 0.000036861190   ,  \"mm2\" -> 0.011651022890   ,  \"mm3\" -> 0.012757340738   ,  \"T\" -> 3.100000000000   ,  \"B\" -> 10.000000000000   ,  \"θ\" -> 45.000000000000   ,  \"Reoff\" -> -204081.632653061300   ,  \"Imoff\" -> 0.000000000000   ,  \"στ1\" -> 0.000238275245   ,  \"στS\" -> 0.000083164391   ,  \"στN\" -> 0.000000428704    |>   , \n\"IDS0490_220602_RAW_cal__sam_\" ->   <|    \"ζ\" -> 0.000000000000   ,  \"τ1\" -> 0.000000000000   ,  \"τS\" -> 0.000000000000   ,  \"τN\" -> 0.000000000000   ,  \"τC\" -> 0.000000000000   ,  \"κ0\" -> 0.000000000000   ,  \"mm1\" -> 0.000000000000   ,  \"mm2\" -> 0.000000000000   ,  \"mm3\" -> 0.000000000000   ,  \"T\" -> 3.100000000000   ,  \"B\" -> 10.000000000000   ,  \"θ\" -> 45.000000000000   ,  \"Reoff\" -> 0.000000000000   ,  \"Imoff\" -> 0.000000000000   ,  \"στ1\" -> 0.000000000000   ,  \"στS\" -> 0.000000000000   ,  \"στN\" -> 0.000000000000    |>   , \n\"IDS0491_220602_RAW_cal__ref_\" ->   <|    \"ζ\" -> 0.018539000460   ,  \"τ1\" -> 0.012513981678   ,  \"τS\" -> 0.005770088680   ,  \"τN\" -> 0.000004734838   ,  \"τC\" -> 0.002222689414   ,  \"κ0\" -> 0.000000055495   ,  \"mm1\" -> 0.000029461735   ,  \"mm2\" -> 0.008061568111   ,  \"mm3\" -> 0.012527524219   ,  \"T\" -> 5.700000000000   ,  \"B\" -> 10.000000000000   ,  \"θ\" -> 45.000000000000   ,  \"Reoff\" -> -69387.755102040828   ,  \"Imoff\" -> 0.000000000000   ,  \"στ1\" -> 0.001996888534   ,  \"στS\" -> 0.001027587268   ,  \"στN\" -> 0.000002006873    |>   , \n\"IDS0491_220602_RAW_cal__sam_\" ->   <|    \"ζ\" -> 0.000000000000   ,  \"τ1\" -> 0.000000000000   ,  \"τS\" -> 0.000000000000   ,  \"τN\" -> 0.000000000000   ,  \"τC\" -> 0.000000000000   ,  \"κ0\" -> 0.000000000000   ,  \"mm1\" -> 0.000000000000   ,  \"mm2\" -> 0.000000000000   ,  \"mm3\" -> 0.000000000000   ,  \"T\" -> 5.700000000000   ,  \"B\" -> 10.000000000000   ,  \"θ\" -> 45.000000000000   ,  \"Reoff\" -> 0.000000000000   ,  \"Imoff\" -> 0.000000000000   ,  \"στ1\" -> 0.000000000000   ,  \"στS\" -> 0.000000000000   ,  \"στN\" -> 0.000000000000    |>   , \n\"IDS0493_220602_RAW_cal__ref_\" ->   <|    \"ζ\" -> 0.240316518824   ,  \"τ1\" -> 0.030134211391   ,  \"τS\" -> 0.077333506670   ,  \"τN\" -> 0.032228870252   ,  \"τC\" -> 0.000888040946   ,  \"κ0\" -> 0.000000000940   ,  \"mm1\" -> 0.000170781534   ,  \"mm2\" -> 0.019820439561   ,  \"mm3\" -> 0.146923057180   ,  \"T\" -> 0.200000000000   ,  \"B\" -> 8.000000000000   ,  \"θ\" -> 45.000000000000   ,  \"Reoff\" -> -33763265.306122481800   ,  \"Imoff\" -> 0.000000000000   ,  \"στ1\" -> 0.022409669919   ,  \"στS\" -> 0.010038141046   ,  \"στN\" -> 0.010969652299    |>   , \n\"IDS0493_220602_RAW_cal__sam_\" ->   <|    \"ζ\" -> 0.000000000000   ,  \"τ1\" -> 0.000000000000   ,  \"τS\" -> 0.000000000000   ,  \"τN\" -> 0.000000000000   ,  \"τC\" -> 0.000000000000   ,  \"κ0\" -> 0.000000000000   ,  \"mm1\" -> 0.000000000000   ,  \"mm2\" -> 0.000000000000   ,  \"mm3\" -> 0.000000000000   ,  \"T\" -> 0.200000000000   ,  \"B\" -> 8.000000000000   ,  \"θ\" -> 45.000000000000   ,  \"Reoff\" -> 0.000000000000   ,  \"Imoff\" -> 0.000000000000   ,  \"στ1\" -> 0.000000000000   ,  \"στS\" -> 0.000000000000   ,  \"στN\" -> 0.000000000000    |>   , \n\"IDS
